vi "Andor DisplayNames.vi"(8 "error in (no error)":errorcluster, 10 "WaveBands":T1(array[cluster]) {"WB End" min=2 max=1024 step=1; "WB Start" min=1 max=1023 step=1}, 11 "numAreas":i32=1) -> (0 "error out":errorcluster, 1 "DatDisplayNm":string[](array[string]))   [LabVIEW 2019]
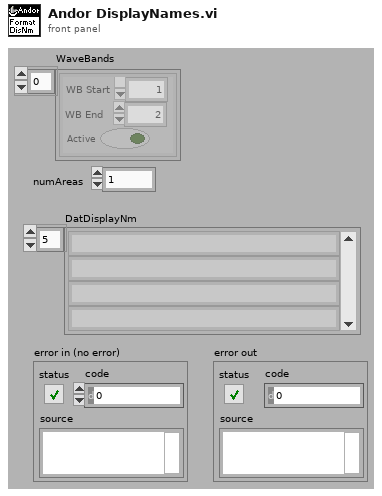
[diagram p1: front panel]
types:
  T1 = cluster{"WB Start":i32, "WB End":i32, "Active":bool}[]
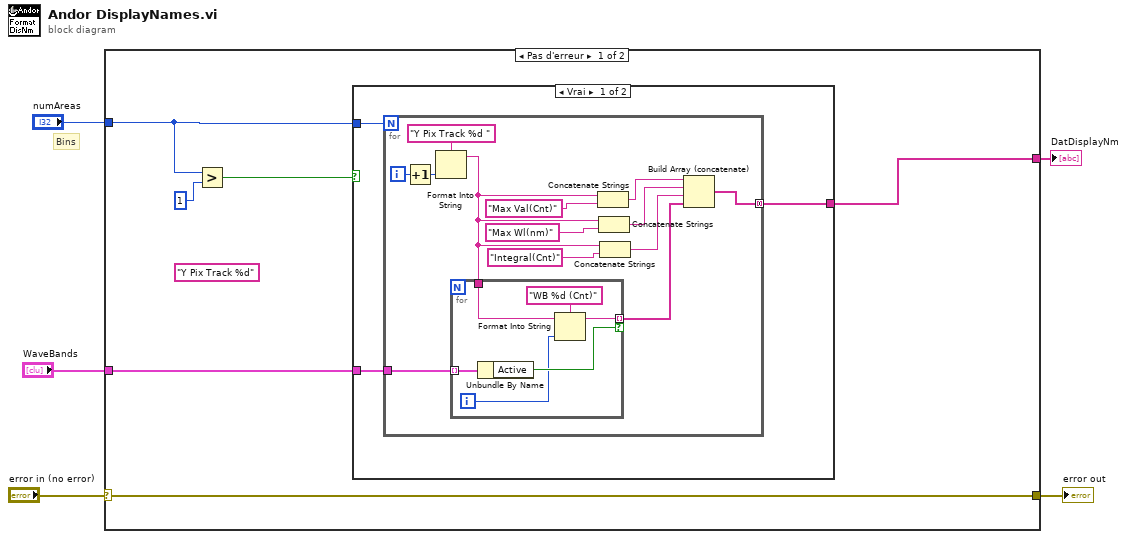
[diagram p0: block diagram]
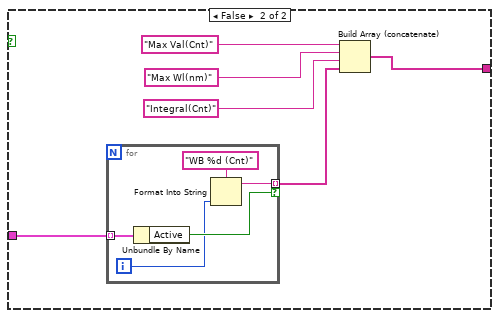
[diagram p2: hidden frame]
diagram:
  # "Bins"
  n1 = case shown="Pas d'erreur" "error in (no error)" {
    selector: "error in (no error)" -> [w11 w45]
    tunnel: "numAreas" -> [w9 _]
    tunnel: [w11 w45] -> w3
    tunnel: [w10 _] -> w2
    tunnel: "WaveBands" -> [w6 _]
    frame No Error {
      (unwired) "Y Pix Track %d"
      n2 = Greater?(x=w9, y=1) -> (0:w7:bool)
      n3 = case shown="Vrai" w7 {
        tunnel: w9 -> [w14 _]
        tunnel: [w13 w39] -> w10
        tunnel: w6 -> [w12 w38]
        frame True {
          n4 = for {
            N: w14 -> [_]
            tunnel: [w26] -> w13 mode=concatenating
            tunnel: w12 -> [w25]
            i -> [w24]
            n5 = Increment(x=w24) -> (x+1=w15:i32)
            n6 = Format Into String(format string="Y Pix Track %d ", w15) -> (resulting string=w17:string)  [unwired: 2 in, 1 out]
            n7 = for {
              tunnel: w25 -> [w32] mode=indexing
              tunnel: w17 -> [w28]
              tunnel: [w31] -> w16 mode=indexing if=w30
              i -> [w29]
              n8 = Unbundle By Name(w32) -> ("Active"=w30:bool)
              n9 = Format Into String(format string="WB %d (Cnt)", initial string=w28, w29) -> (resulting string=w31:string)  [unwired: 1 in, 1 out]
            }
            n10 = Concatenate Strings(w17, "Max Val(Cnt)") -> (w20:string)
            n11 = Concatenate Strings(w17, "Max Wl(nm)") -> (w19:string)
            n12 = Concatenate Strings(w17, "Integral(Cnt)") -> (w18:string)
            n13 = Build Array (concatenate)(w20, w19, w18, w16) -> (w26:string[])
          }
        }
        frame False {
          n14 = for {
            tunnel: w38 -> [w43] mode=indexing
            tunnel: [w42] -> w37 mode=indexing if=w41
            i -> [w40]
            n15 = Unbundle By Name(w43) -> ("Active"=w41:bool)
            n16 = Format Into String(format string="WB %d (Cnt)", w40) -> (resulting string=w42:string)  [unwired: 2 in, 1 out]
          }
          n17 = Build Array (concatenate)("Max Val(Cnt)", "Max Wl(nm)", "Integral(Cnt)", w37) -> (w39:string[])
        }
      }
    }
    frame Error {
    }
  }
  "error out" <- w3
  "DatDisplayNm" <- w2
